vi "HovaCAL ppm convert from Component.vi"(10 "Konzentration":dbl, 11 "Gasnummer":T2) -> (0 "Komponenten Name":T1, 1 "Konzentration in ppm":dbl, 2 "Konzentration in %":dbl, 3 "Gasnummer out":T2, 5 "Einheit in String":string)   [LabVIEW 2020, in "Linearisierung v2.lvlib" / "Gasteiler.lvlib" / "HovaCAL_Interface.lvlib" / "Helper.lvlib"]
uses:
  Helper.lvlib
  Visualisierungs Elemente/Auswahlfeld.ctl
  Visualisierungs Elemente/String - Ausgabefeld.ctl
  Gasteiler.lvlib
  SpanEinstellungen/SpanEinstellungen.lvlib
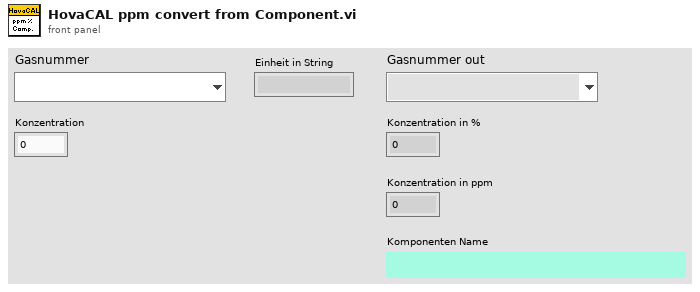
[diagram p1: front panel]
types:
  T1 = typedef "String - Ausgabefeld.ctl" = string
  T2 = typedef "Auswahlfeld.ctl" = u16
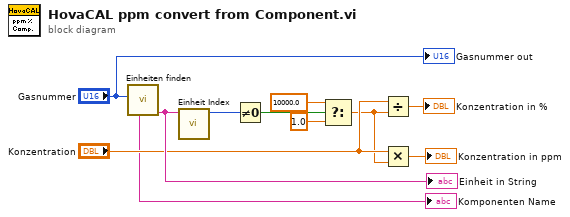
[diagram p0: block diagram]
diagram:
  n1 = call "Einheiten finden.vi"("Komponente"="Gasnummer") -> ("Einheit in String"=w5:string, "Komponenten Name"=→"Komponenten Name":T1)  [unwired: 6 in, 3 out]
  "Einheit in String" <- w5
  n2 = call "Einheit Index.vi"("Einheit in String"=w5) -> ("Elementindex"=w6:i32)  [unwired: 10 in]
  n3 = Not Equal To 0?(x=w6) -> (x != 0?=w9:bool)
  n4 = Select(t=10000.0 ("y"), s=w9, f=1.0) -> (s? t:f=w3:dbl)
  n5 = Divide(x="Konzentration", y=w3) -> (x/y=→"Konzentration in %":dbl)
  n6 = Multiply(x="Konzentration", y=w3) -> (x*y=→"Konzentration in ppm":dbl)
  "Gasnummer out" <- "Gasnummer"
